vi "findText.vi"(8 "Error In":errorcluster, 9 "flags":T1 items=["MatchExactly"=0, "MatchContains"=1, "MatchStartsWith"=2, "MatchEndsWith"=3, "MatchRegExp"=4, "MatchWildcard"=5, "MatchFixedString"=8, "MatchCaseSensitive"=16, "MatchWrap"=32, "MatchRecursive"=64], 10 "text":string, 11 "QComboBox In":refnum<class "QComboBox.lvclass">) -> (0 "Error Out":errorcluster, 2 "Value":i32, 3 "QComboBox Out":refnum<class "QComboBox.lvclass">)   [LabVIEW 2014, in "QComboBox.lvclass"]
doc: "LabVIEW-specific documentation is not yet available. See <b>https://doc.qt.io/qt-5/qcombobox.html#findText</b>"
uses:
  QComboBox.lvclass
  LQ Core/Qt/MatchFlag.ctl
  LQ Core/LQIdentity/LQIdentity.lvclass/LQIdentity.ctl
  LQ Core/LQ Core.lvlib
  LQ Core/LQIdentity/LQIdentity.lvclass
  LQ Core/Qt/Qt.lvlib
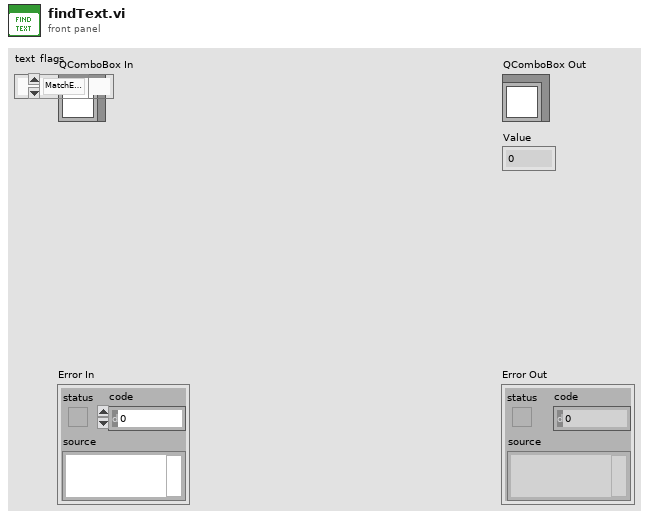
[diagram p1: front panel]
types:
  T1 = typedef "Qt.lvlib/MatchFlag.ctl" = i32
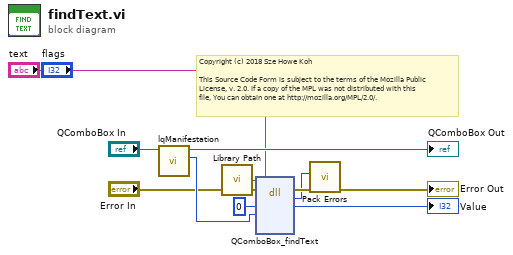
[diagram p0: block diagram]
diagram:
  # "Copyright (c) 2018 Sze Howe Koh\n\nThis Source Code Form is subject to the terms of the Mozilla Public\nLicense, v. 2.0. If a copy of the MPL was not distributed with this\nfile, You can obtain one at http://mozilla.org/MPL/2.0/."
  n1 = call "lqManifestation.vi"("LQIdentity in"="QComboBox In") -> ("Manifestation"=w7:u64, "LQIdentity out"=→"QComboBox Out":refnum<class "QComboBox.lvclass">)  [unwired: 9 in]
  n2 = call "Library Path.vi"() -> ("Library Path"=w8:path)
  n3 = dll-call lib="?" fn="QComboBox_findText"(path in=w8, error in="Error In", "_retVal"=0 ("retVal"), "_instance"=w7, "text"="text", "flags"="flags") -> (error out=w5:errorcluster, w3:i32, "_retVal"=→"Value":i32)  [unwired: 4 in, 1 out]
  n4 = call "Pack Errors.vi"("Error In"=w5, "Error Code"=w3) -> ("Error Out"=→"Error Out":errorcluster)  [unwired: 9 in]
